vi "读写配置文件.vi"(8 "BoardConfig_input":T1, 10 "文件名称":string, 11 "m_bRead":bool) -> (2 "BoardConfig_output":T1)   [LabVIEW 2010]
doc: "读写以太网配置文件\n\n参数 m_bRead：\nTRUE 为读配置 FALSE 为写配置\n\n参数 io_put_write：\n当 m_bRead 为 FALSE 写配置时 如果该值为 0 表示写输入配置 1 表示写输出配置"
uses:
  <vilib>/Utility/config.llb/Write Key (I32).vi
  <vilib>/Utility/config.llb/Write Key (U32).vi
  <vilib>/Utility/config.llb/Write Key (Double).vi
  <vilib>/Utility/config.llb/Write Key (Boolean).vi
  <vilib>/Utility/config.llb/Write Key (String).vi
  <vilib>/Utility/config.llb/Read Key (U32).vi
  <vilib>/Utility/config.llb/Read Key (Double).vi
  <vilib>/Utility/config.llb/Read Key (I32).vi
  <vilib>/Utility/config.llb/Read Key (Boolean).vi
  <vilib>/Utility/config.llb/Read Key (String).vi
  <vilib>/Utility/config.llb/NI_LVConfig.lvlib
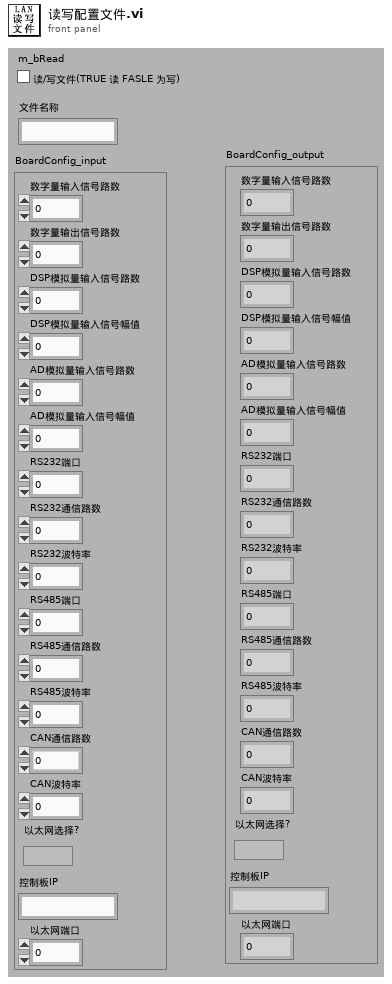
[diagram p1: front panel]
types:
  T1 = cluster{"数字量输入信号路数":i32, "数字量输出信号路数":i32, "DSP模拟量输入信号路数":u32, "DSP模拟量输入信号幅值":u32, "AD模拟量输入信号路数":u32, "AD模拟量输入信号幅值":u32, "RS232端口":u32, "RS232通信路数":u32, "RS232波特率":dbl, "RS485端口":u32, "RS485通信路数":u32, "RS485波特率":u32, "CAN通信路数":i32, "CAN波特率":u32, "以太网选择?":bool, "控制板IP":string, "以太网端口":u32}
  T2 = typedef "NI_LVConfig.lvlib/Config Data RefNum.ctl" = refnum<k1>
  T3 = cluster{"value":u32, "value":u32, "value":u32, "value":u32, "value":u32, "value":u32, "value":u32, "value":u32, "value":dbl, "value":u32, "value":u32, "value":u32, "value":i32, "value":u32, "value":bool, "value":string, "value":u32}
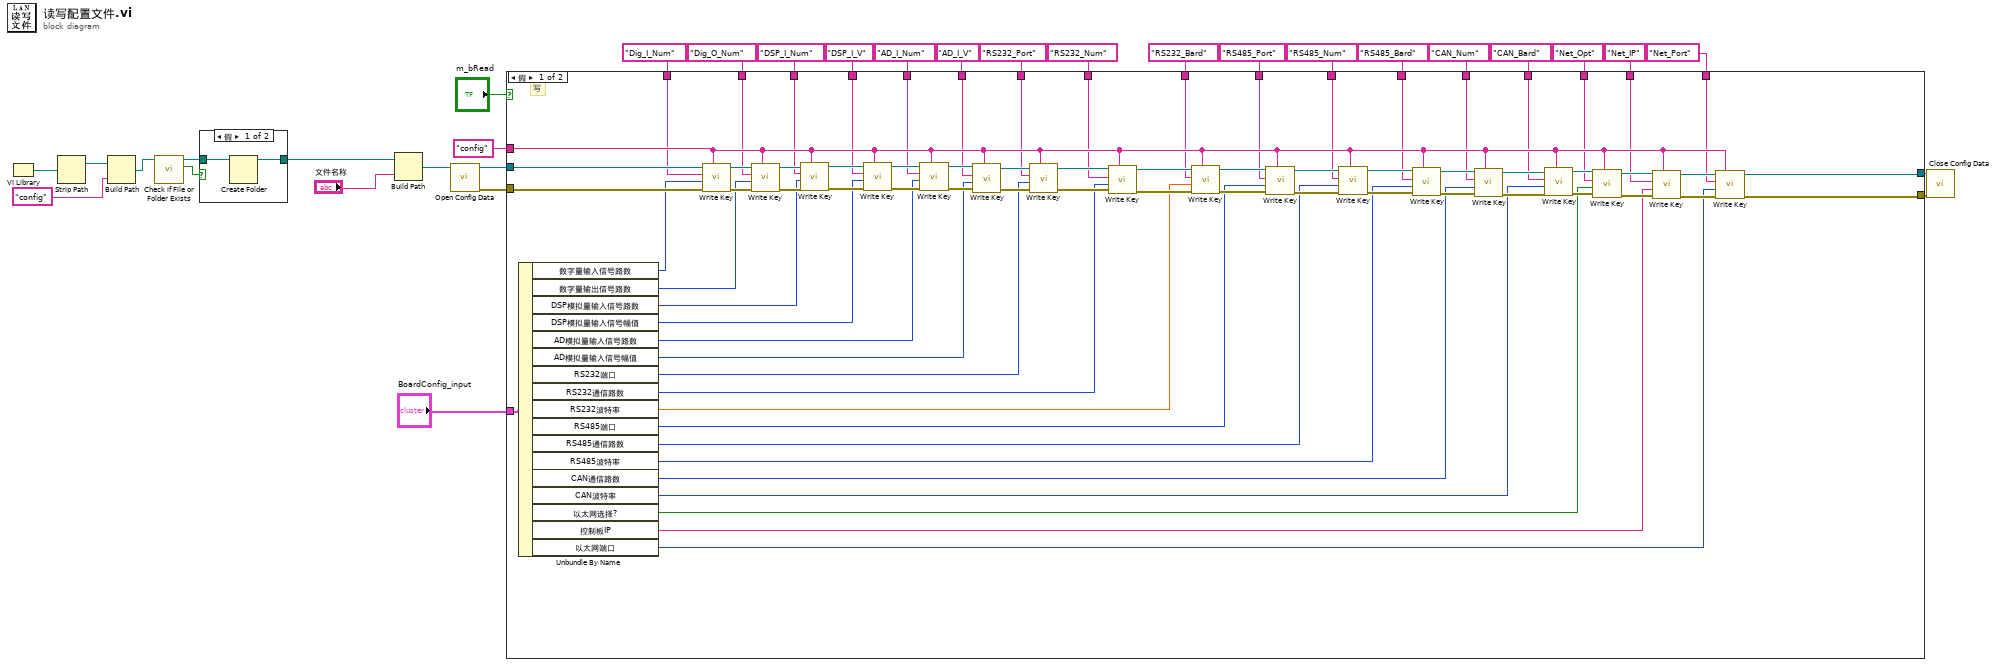
[diagram p0: block diagram]
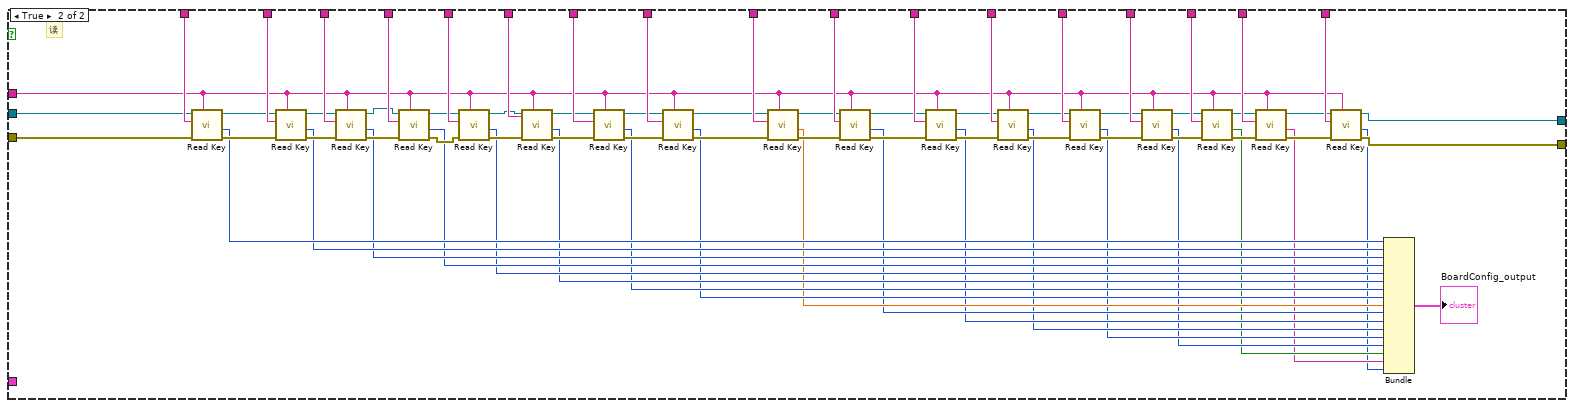
[diagram p2: hidden frame]
diagram:
  n1 = VI Library() -> (path=w32:path)
  n2 = Strip Path(path=w32) -> (stripped path=w33:path)  [unwired: 1 out]
  n3 = Build Path(base path=w33, name or relative path="config") -> (appended path=w30:path)
  n4 = call <vilib>:"Check if File or Folder Exists.vi"("path"=w30) -> ("file or folder exists?"=w29:bool, "dup path"=w28:path)  [unwired: 8 in, 1 out]
  n5 = case shown="假" w29 {
    tunnel: w28 -> [w34 w36]
    tunnel: [w35 w36] -> w20
    frame False {
      n6 = Create Folder(path (use dialog)=w34) -> (created path=w35:path)  [unwired: 2 in, 2 out]
    }
    frame True {
    }
  }
  n7 = Build Path(base path=w20, name or relative path="文件名称") -> (appended path=w27:path)
  n8 = call <vilib>:"Open Config Data.vi"("configuration file path"=w27) -> ("error out"=w24:errorcluster, "refnum"=w25:T2)  [unwired: 8 in, 1 out]
  n9 = case shown="假" "m_bRead" {
    tunnel: w25 -> [w108 w163]
    tunnel: w24 -> [w107 w162]
    tunnel: "config" -> [w62 w127]
    tunnel: [w64 w139] -> w22
    tunnel: [w63 w128] -> w21
    tunnel: "BoardConfig_input" -> [w104 _]
    tunnel: "Dig_I_Num" ("key") -> [w53 w180]
    tunnel: "Dig_O_Num" ("key") -> [w52 w179]
    tunnel: "DSP_I_Num" ("key") -> [w51 w178]
    tunnel: "DSP_I_V" ("key") -> [w50 w177]
    tunnel: "AD_I_Num" ("key") -> [w49 w176]
    tunnel: "AD_I_V" ("key") -> [w48 w175]
    tunnel: "RS232_Port" ("key") -> [w47 w174]
    tunnel: "RS232_Num" ("key") -> [w46 w173]
    tunnel: "RS232_Bard" ("key") -> [w45 w172]
    tunnel: "RS485_Port" ("key") -> [w44 w171]
    tunnel: "RS485_Num" ("key") -> [w43 w170]
    tunnel: "RS485_Bard" ("key") -> [w42 w169]
    tunnel: "CAN_Num" ("key") -> [w41 w168]
    tunnel: "CAN_Bard" ("key") -> [w40 w167]
    tunnel: "Net_Opt" ("key") -> [w39 w166]
    tunnel: "Net_IP" ("key") -> [w38 w165]
    tunnel: "Net_Port" ("key") -> [w37 w164]
    frame False {
      # "写"
      n10 = Unbundle By Name(w104) -> ("数字量输入信号路数"=w103:i32, "数字量输出信号路数"=w100:i32, "DSP模拟量输入信号路数"=w97:u32, "DSP模拟量输入信号幅值"=w94:u32, "AD模拟量输入信号路数"=w93:u32, "AD模拟量输入信号幅值"=w90:u32, "RS232端口"=w87:u32, "RS232通信路数"=w82:u32, "RS232波特率"=w81:dbl, "RS485端口"=w61:u32, "RS485通信路数"=w60:u32, "RS485波特率"=w59:u32, "CAN通信路数"=w58:i32, "CAN波特率"=w57:u32, "以太网选择?"=w56:bool, "控制板IP"=w55:string, "以太网端口"=w54:u32)
      n11 = call-poly <vilib>:"Write Key.vi"("section"=w62, "error in (no error)"=w107, "value"=w103, "key"=w53, "refnum"=w108) -> ("error out"=w101:errorcluster, "refnum out"=w102:T2)  [unwired: 4 in, 1 out]
      n12 = call-poly <vilib>:"Write Key.vi"("section"=w62, "error in (no error)"=w101, "value"=w100, "key"=w52, "refnum"=w102) -> ("error out"=w98:errorcluster, "refnum out"=w99:T2)  [unwired: 4 in, 1 out]
      n13 = call-poly <vilib>:"Write Key.vi"("section"=w62, "error in (no error)"=w98, "value"=w97, "key"=w51, "refnum"=w99) -> ("error out"=w95:errorcluster, "refnum out"=w96:T2)  [unwired: 4 in, 1 out]
      n14 = call-poly <vilib>:"Write Key.vi"("section"=w62, "error in (no error)"=w95, "value"=w94, "key"=w50, "refnum"=w96) -> ("error out"=w105:errorcluster, "refnum out"=w106:T2)  [unwired: 4 in, 1 out]
      n15 = call-poly <vilib>:"Write Key.vi"("section"=w62, "error in (no error)"=w105, "value"=w93, "key"=w49, "refnum"=w106) -> ("error out"=w91:errorcluster, "refnum out"=w92:T2)  [unwired: 4 in, 1 out]
      n16 = call-poly <vilib>:"Write Key.vi"("section"=w62, "error in (no error)"=w91, "value"=w90, "key"=w48, "refnum"=w92) -> ("error out"=w89:errorcluster, "refnum out"=w88:T2)  [unwired: 4 in, 1 out]
      n17 = call-poly <vilib>:"Write Key.vi"("section"=w62, "error in (no error)"=w89, "value"=w87, "key"=w47, "refnum"=w88) -> ("error out"=w86:errorcluster, "refnum out"=w85:T2)  [unwired: 4 in, 1 out]
      n18 = call-poly <vilib>:"Write Key.vi"("section"=w62, "error in (no error)"=w86, "value"=w82, "key"=w46, "refnum"=w85) -> ("error out"=w83:errorcluster, "refnum out"=w84:T2)  [unwired: 4 in, 1 out]
      n19 = call-poly <vilib>:"Write Key.vi"("section"=w62, "error in (no error)"=w83, "value"=w81, "key"=w45, "refnum"=w84) -> ("error out"=w76:errorcluster, "refnum out"=w77:T2)  [unwired: 4 in, 1 out]
      n20 = call-poly <vilib>:"Write Key.vi"("section"=w62, "error in (no error)"=w76, "value"=w61, "key"=w44, "refnum"=w77) -> ("error out"=w75:errorcluster, "refnum out"=w78:T2)  [unwired: 4 in, 1 out]
      n21 = call-poly <vilib>:"Write Key.vi"("section"=w62, "error in (no error)"=w75, "value"=w60, "key"=w43, "refnum"=w78) -> ("error out"=w73:errorcluster, "refnum out"=w74:T2)  [unwired: 4 in, 1 out]
      n22 = call-poly <vilib>:"Write Key.vi"("section"=w62, "error in (no error)"=w73, "value"=w59, "key"=w42, "refnum"=w74) -> ("error out"=w71:errorcluster, "refnum out"=w72:T2)  [unwired: 4 in, 1 out]
      n23 = call-poly <vilib>:"Write Key.vi"("section"=w62, "error in (no error)"=w71, "value"=w58, "key"=w41, "refnum"=w72) -> ("error out"=w79:errorcluster, "refnum out"=w80:T2)  [unwired: 4 in, 1 out]
      n24 = call-poly <vilib>:"Write Key.vi"("section"=w62, "error in (no error)"=w79, "value"=w57, "key"=w40, "refnum"=w80) -> ("error out"=w69:errorcluster, "refnum out"=w70:T2)  [unwired: 4 in, 1 out]
      n25 = call-poly <vilib>:"Write Key.vi"("section"=w62, "error in (no error)"=w69, "value"=w56, "key"=w39, "refnum"=w70) -> ("error out"=w67:errorcluster, "refnum out"=w68:T2)  [unwired: 4 in, 1 out]
      n26 = call-poly <vilib>:"Write Key.vi"("section"=w62, "error in (no error)"=w67, "value"=w55, "key"=w38, "refnum"=w68) -> ("error out"=w65:errorcluster, "refnum out"=w66:T2)  [unwired: 4 in, 1 out]
      n27 = call-poly <vilib>:"Write Key.vi"("section"=w62, "error in (no error)"=w65, "value"=w54, "key"=w37, "refnum"=w66) -> ("error out"=w63:errorcluster, "refnum out"=w64:T2)  [unwired: 4 in, 1 out]
    }
    frame True {
      # "读"
      n28 = call-poly <vilib>:"Read Key.vi"("section"=w127, "error in (no error)"=w162, "key"=w180, "refnum"=w163) -> ("error out"=w160:errorcluster, "value"=w126:u32, "refnum out"=w161:T2)  [unwired: 4 in, 1 out]
      n29 = call-poly <vilib>:"Read Key.vi"("section"=w127, "error in (no error)"=w160, "key"=w179, "refnum"=w161) -> ("error out"=w158:errorcluster, "value"=w125:u32, "refnum out"=w159:T2)  [unwired: 4 in, 1 out]
      n30 = call-poly <vilib>:"Read Key.vi"("section"=w127, "error in (no error)"=w158, "key"=w178, "refnum"=w159) -> ("error out"=w156:errorcluster, "value"=w124:u32, "refnum out"=w157:T2)  [unwired: 4 in, 1 out]
      n31 = call-poly <vilib>:"Read Key.vi"("section"=w127, "error in (no error)"=w156, "key"=w177, "refnum"=w157) -> ("error out"=w154:errorcluster, "value"=w123:u32, "refnum out"=w155:T2)  [unwired: 4 in, 1 out]
      n32 = call-poly <vilib>:"Read Key.vi"("section"=w127, "error in (no error)"=w154, "key"=w176, "refnum"=w155) -> ("error out"=w152:errorcluster, "value"=w122:u32, "refnum out"=w153:T2)  [unwired: 4 in, 1 out]
      n33 = call-poly <vilib>:"Read Key.vi"("section"=w127, "error in (no error)"=w152, "key"=w175, "refnum"=w153) -> ("error out"=w150:errorcluster, "value"=w121:u32, "refnum out"=w151:T2)  [unwired: 4 in, 1 out]
      n34 = call-poly <vilib>:"Read Key.vi"("section"=w127, "error in (no error)"=w150, "key"=w174, "refnum"=w151) -> ("error out"=w138:errorcluster, "value"=w120:u32, "refnum out"=w149:T2)  [unwired: 4 in, 1 out]
      n35 = call-poly <vilib>:"Read Key.vi"("section"=w127, "error in (no error)"=w138, "key"=w173, "refnum"=w149) -> ("error out"=w137:errorcluster, "value"=w119:u32, "refnum out"=w148:T2)  [unwired: 4 in, 1 out]
      n36 = call-poly <vilib>:"Read Key.vi"("section"=w127, "error in (no error)"=w137, "key"=w172, "refnum"=w148) -> ("error out"=w136:errorcluster, "value"=w118:dbl, "refnum out"=w147:T2)  [unwired: 4 in, 1 out]
      n37 = call-poly <vilib>:"Read Key.vi"("section"=w127, "error in (no error)"=w136, "key"=w171, "refnum"=w147) -> ("error out"=w135:errorcluster, "value"=w117:u32, "refnum out"=w146:T2)  [unwired: 4 in, 1 out]
      n38 = call-poly <vilib>:"Read Key.vi"("section"=w127, "error in (no error)"=w135, "key"=w170, "refnum"=w146) -> ("error out"=w134:errorcluster, "value"=w116:u32, "refnum out"=w145:T2)  [unwired: 4 in, 1 out]
      n39 = call-poly <vilib>:"Read Key.vi"("section"=w127, "error in (no error)"=w134, "key"=w169, "refnum"=w145) -> ("error out"=w133:errorcluster, "value"=w115:u32, "refnum out"=w144:T2)  [unwired: 4 in, 1 out]
      n40 = call-poly <vilib>:"Read Key.vi"("section"=w127, "error in (no error)"=w133, "key"=w168, "refnum"=w144) -> ("error out"=w132:errorcluster, "value"=w114:i32, "refnum out"=w143:T2)  [unwired: 4 in, 1 out]
      n41 = call-poly <vilib>:"Read Key.vi"("section"=w127, "error in (no error)"=w132, "key"=w167, "refnum"=w143) -> ("error out"=w131:errorcluster, "value"=w113:u32, "refnum out"=w142:T2)  [unwired: 4 in, 1 out]
      n42 = call-poly <vilib>:"Read Key.vi"("section"=w127, "error in (no error)"=w131, "key"=w166, "refnum"=w142) -> ("error out"=w130:errorcluster, "value"=w112:bool, "refnum out"=w141:T2)  [unwired: 4 in, 1 out]
      n43 = call-poly <vilib>:"Read Key.vi"("section"=w127, "error in (no error)"=w130, "key"=w165, "refnum"=w141) -> ("error out"=w129:errorcluster, "value"=w111:string, "refnum out"=w140:T2)  [unwired: 4 in, 1 out]
      n44 = call-poly <vilib>:"Read Key.vi"("section"=w127, "error in (no error)"=w129, "key"=w164, "refnum"=w140) -> ("error out"=w128:errorcluster, "value"=w110:u32, "refnum out"=w139:T2)  [unwired: 4 in, 1 out]
      n45 = Bundle("value"=w126, "value"=w125, "value"=w124, "value"=w123, "value"=w122, "value"=w121, "value"=w120, "value"=w119, "value"=w118, "value"=w117, "value"=w116, "value"=w115, "value"=w114, "value"=w113, "value"=w112, "value"=w111, "value"=w110) -> (→"BoardConfig_output":T3)  [unwired: 1 in]
    }
  }
  n46 = call <vilib>:"Close Config Data.vi"("error in (no error)"=w21, "refnum"=w22) -> ()  [unwired: 8 in, 2 out]
